vi "Decorate.vi"(8 "error in (no error)":errorcluster, 10 "Component":refnum<class "Component.lvclass">, 11 "Decorator in":refnum<class "Decorator.lvclass">) -> (0 "error out":errorcluster, 3 "Decorator out":refnum<class "Decorator.lvclass">)   [LabVIEW 2014, in "Decorator.lvclass"]
uses:
  Decorator.lvclass
  Component_class/Component.lvclass
  Decorator.lvclass/Decorator.ctl
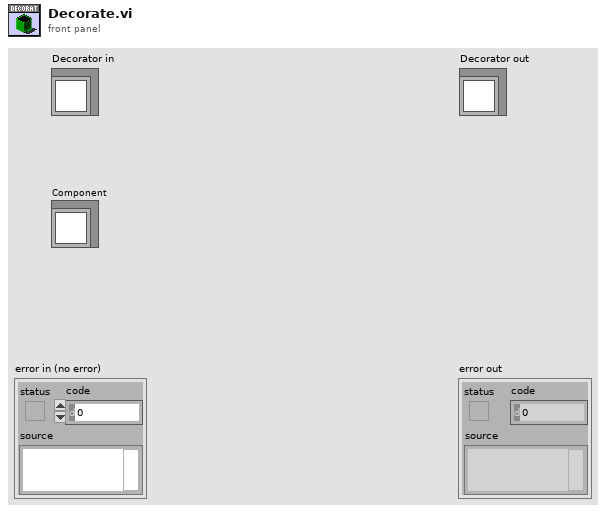
[diagram p1: front panel]
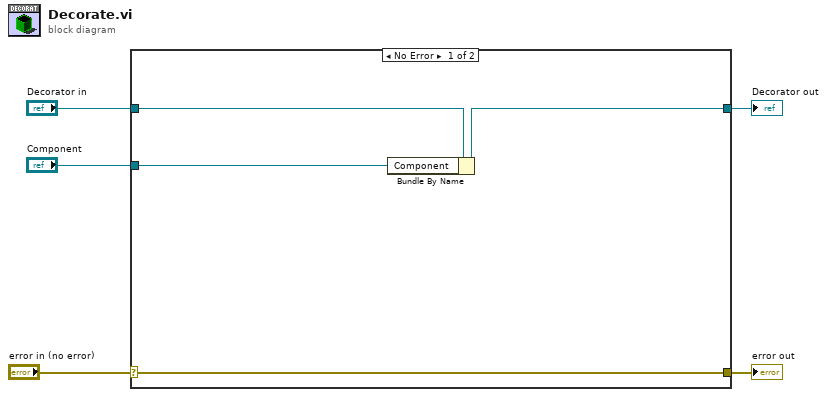
[diagram p0: block diagram]
diagram:
  n1 = case shown="No Error" "error in (no error)" {
    selector: "error in (no error)" -> [w8 w11]
    tunnel: [w8 w11] -> w4
    tunnel: [w7 w10] -> w2
    tunnel: "Decorator in" -> [w9 w10]
    tunnel: "Component" -> [w6 _]
    frame No Error {
      n2 = Bundle By Name(cluster=w9, "Component"=w6) -> (w7:refnum<class "Decorator.lvclass">)
    }
    frame Error {
    }
  }
  "error out" <- w4
  "Decorator out" <- w2
